vi "My Globals.vi"() -> ()   [LabVIEW 2015]
panel:
  in  "Sine values":dbl
  in  "start":bool
  in  "stop":bool
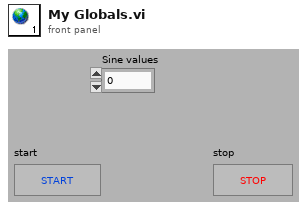
[diagram p1: front panel]
diagram:
